vi "InitState.vi"(9 "Container State":T2, 11 "Control State in":T1) -> (3 "Control State out":T1)   [LabVIEW 2019, in "ExpandVertical.xctl"]
uses:
  ExpandVertical.xctl
  <vilib>/_xctls/Container State.ctl
  State.ctl
  <vilib>/_xctls/XControlSupport.lvlib
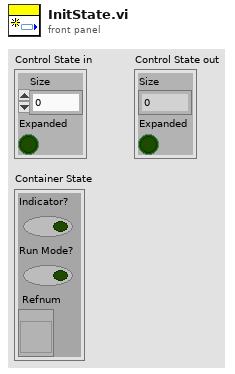
[diagram p1: front panel]
types:
  T1 = typedef "ExpandVertical.xctl/State.ctl" = cluster{"Size":i16, "Expanded":bool}
  T2 = typedef "XControlSupport.lvlib/Container State.ctl" = cluster{"Indicator?":bool, "Run Mode?":bool, " Refnum":refnum<vi>}
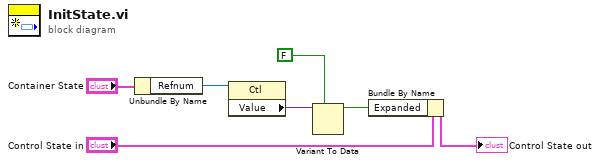
[diagram p0: block diagram]
diagram:
  n1 = Unbundle By Name("Container State") -> ("Refnum"=w5:refnum<vi>)
  n2 = property class="Ctl"(reference=w5) -> ("Value"=w4:variant)  [unwired: 1 in, 2 out]
  n3 = Variant To Data(type=FALSE, Variant=w4) -> (data=w1:bool)  [unwired: 1 in, 1 out]
  n4 = Bundle By Name(cluster="Control State in", "Expanded"=w1) -> (→"Control State out":T1)
